vi "Mux2.vi"   [LabVIEW 2019]
uses:
  <vilib>/eio/EIOGrowableMethodNode/genericMethod/EIOGrowableMethodNode.xnode
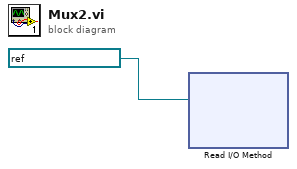
[diagram p0: block diagram]
diagram:
  n1 = xnode "Read I/O Method"("FPGA I/O In"=refnum<k21> "Connector0/AI0") -> ()  [unwired: 2 in, 4 out]
